vi "PythonSessionFGV.vi"(8 "error in":errorcluster, 10 "state":string(combo)="close") -> (0 "error out":errorcluster, 2 "PythonSession":refnum<k35>)   [LabVIEW 2020]
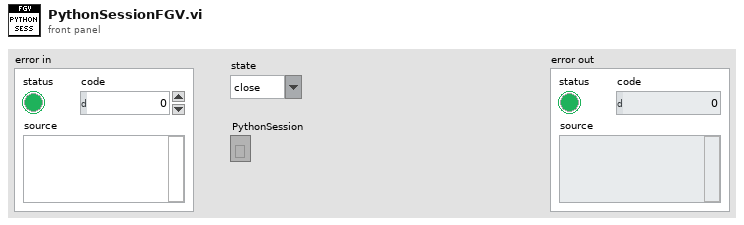
[diagram p1: front panel]
types:
  T1 = cluster{"PythonSession":refnum<k35>, "session_open":bool}
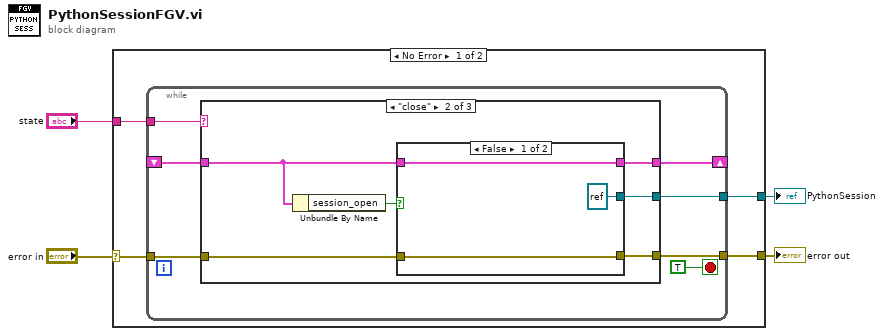
[diagram p0: block diagram]
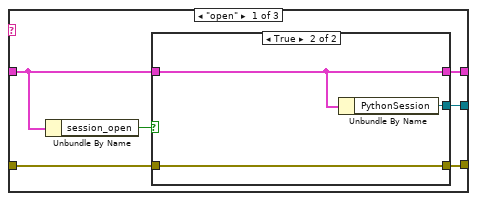
[diagram p2: hidden frame]
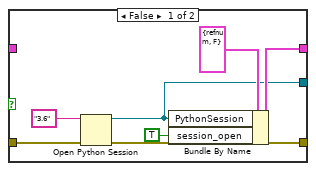
[diagram p3: hidden frame]
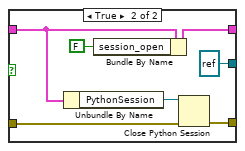
[diagram p4: hidden frame]
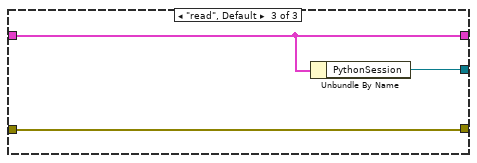
[diagram p5: hidden frame]
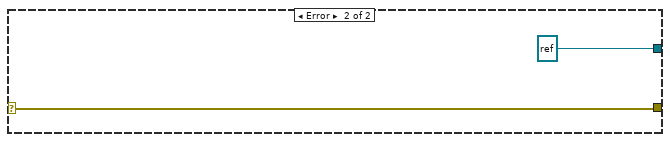
[diagram p6: hidden frame]
diagram:
  n1 = case shown="No Error" "error in" {
    selector: "error in" -> [w8 w51]
    tunnel: "state" -> [w7 _]
    tunnel: [w6 w51] -> w2
    tunnel: [w5 refnum<k35> refnum ("PythonSession")] -> w1
    frame No Error {
      n2 = while {
        tunnel: w8 -> [w14]
        tunnel: w7 -> [w13]
        shift-right: [w12] -> _
        shift-left: _ -> [w10]
        tunnel: [w11] -> w6
        tunnel: [w9] -> w5
        stop <- TRUE stop-if-true
        n3 = case shown="\"close\"" w13 {
          tunnel: w14 -> [w21 w37 w48]
          tunnel: [w20 w35 w50] -> w12
          tunnel: [w19 w36 w48] -> w11
          tunnel: w10 -> [w16 w33 w50]
          tunnel: [w18 w34 w49] -> w9
          frame "open" {
            n4 = Unbundle By Name(w16) -> ("session_open"=w17:bool)
            n5 = case shown="True" w17 {
              tunnel: w21 -> [w27 w29]
              tunnel: [w24 w31] -> w20
              tunnel: [w23 w29] -> w19
              tunnel: [w22 w30] -> w18
              tunnel: w16 -> [_ w31]
              frame False {
                n6 = Open Python Session(python version="3.6" ("Python version"), 3:w27) -> (session out=w22:refnum<k35>, error out=w23:errorcluster)  [unwired: 1 in]
                n7 = Bundle By Name(cluster=T1 {"PythonSession"=refnum, "session_open"=FALSE} ("Local"), "PythonSession"=w22, "session_open"=TRUE) -> (w24:T1)
              }
              frame True {
                n8 = Unbundle By Name(w31) -> ("PythonSession"=w30:refnum<k35>)
              }
            }
          }
          frame "close" {
            n9 = Unbundle By Name(w33) -> ("session_open"=w32:bool)
            n10 = case shown="False" w32 {
              tunnel: w37 -> [w38 w46]
              tunnel: [w38 w45] -> w36
              tunnel: w33 -> [w40 w44]
              tunnel: [w40 w42] -> w35
              tunnel: [refnum<k35> refnum ("PythonSession") refnum<k35> refnum ("PythonSession")] -> w34
              frame False {
              }
              frame True {
                n11 = Unbundle By Name(w44) -> ("PythonSession"=w47:refnum<k35>)
                n12 = Bundle By Name(cluster=w44, "session_open"=FALSE) -> (w42:T1)
                n13 = Close Python Session(session in=w47, error in=w46) -> (11:w45:errorcluster)
              }
            }
          }
          frame "read", Default {
            n14 = Unbundle By Name(w50) -> ("PythonSession"=w49:refnum<k35>)
          }
        }
      }
    }
    frame Error {
    }
  }
  "error out" <- w2
  "PythonSession" <- w1
